vi "Write 2DPictureRef.vi"(8 "error in (no error)":errorcluster, 10 "2DPictureRef":refnum<vi>, 11 "2DPictureControl in":refnum<class "2DPictureControl.lvclass">=refnum) -> (0 "error out":errorcluster, 3 "2DPictureControl out":refnum<class "2DPictureControl.lvclass">)   [LabVIEW 2020, in "2DPictureControl.lvclass"]
uses:
  2DPictureControl.lvclass
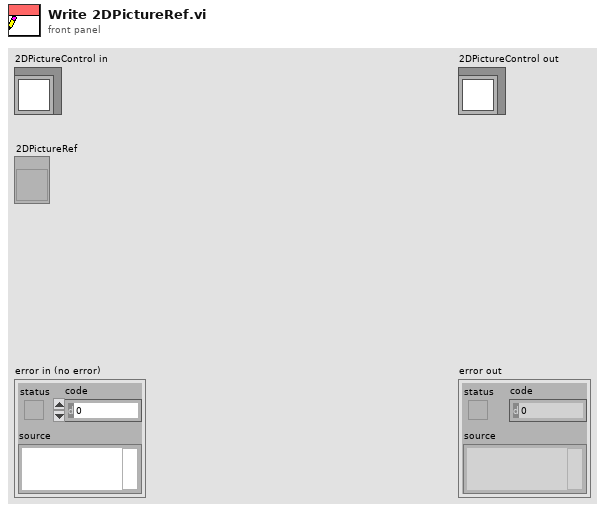
[diagram p1: front panel]
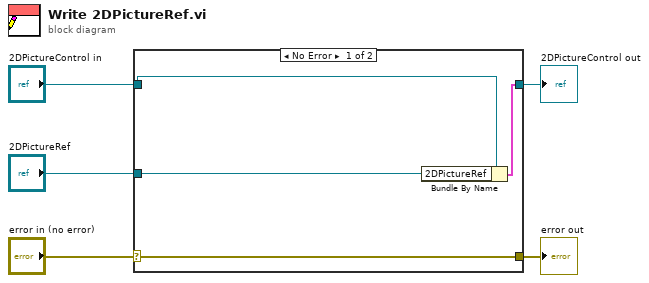
[diagram p0: block diagram]
diagram:
  n1 = case shown="No Error" "error in (no error)" {
    selector: "error in (no error)" -> [w9 w10]
    tunnel: [w9 w10] -> w4
    tunnel: [w7 w11] -> w2
    tunnel: "2DPictureControl in" -> [w8 w11]
    tunnel: "2DPictureRef" -> [w6 _]
    frame No Error {
      n2 = Bundle By Name(cluster=w8, "2DPictureRef"=w6) -> (w7:cluster{})
    }
    frame Error {
    }
  }
  "error out" <- w4
  "2DPictureControl out" <- w2
